vi "aproximateBall.vi"(6 "Radius":dbl, 8 "error in (no error)":errorcluster, 9 "Ball":refnum<class "Ball.lvclass">, 10 "Robot":refnum<class "Robot.lvclass">, 11 "KickToSkill in":refnum<class "KickToSkill.lvclass">) -> (0 "error out":errorcluster, 2 "Robot out":refnum<class "Robot.lvclass">, 3 "KickToSkill out":refnum<class "KickToSkill.lvclass">)   [LabVIEW 2023, in "KickToSkill.lvclass"]
uses:
  KickToSkill.lvclass
  Ball_class/Ball.lvclass
  C:/Users/lucio/Desktop/roboime/SSL_AI/Object_class/Object.lvclass
  Robot_class/Robot.lvclass
  Object_class/Object.lvclass/Object.ctl
  Robot_class/Robot.lvclass/Robot.ctl
  <vilib>/Analysis/baseanly.llb/Unit Vector (DBL).vi
  Object_class/Read position(x,y).vi
  Robot_class/Write dest_x.vi
  Robot_class/Write dest_y.vi
  Robot_class/Write dest_orientation.vi
  Utilities_class/Utilities.lvclass
  <vilib>/Analysis/NI_AALBase.lvlib
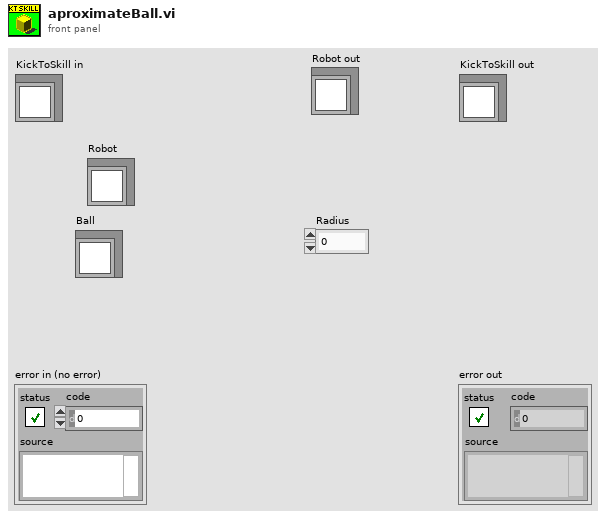
[diagram p1: front panel]
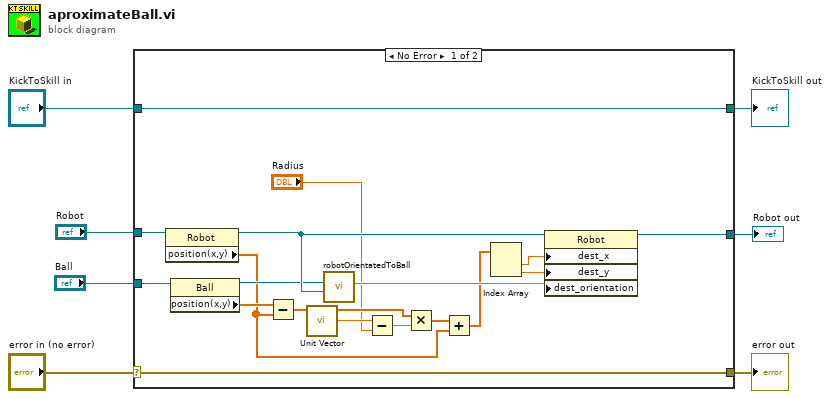
[diagram p0: block diagram]
diagram:
  n1 = case shown="No Error" "error in (no error)" {
    selector: "error in (no error)" -> [w25 w29]
    tunnel: [w25 w29] -> w6
    tunnel: [w26 w28] -> w4
    tunnel: "KickToSkill in" -> [w26 w28]
    tunnel: "Robot" -> [w23 w27]
    tunnel: "Ball" -> [w21 _]
    tunnel: [w9 w27] -> w1
    frame No Error {
      n2 = property class="Robot"(reference=w23) -> (reference out=w22:refnum<class "Robot.lvclass">, "position(x,y)"=w13:dbl[])  [unwired: 1 in, 1 out]
      n3 = property class="Ball"(reference=w21) -> (reference out=w20:refnum<class "Ball.lvclass">, "position(x,y)"=w19:dbl[])  [unwired: 1 in, 1 out]
      n4 = Subtract(x=w19, y=w13) -> (x-y=w18:dbl[])
      n5 = call-poly <vilib>:"Unit Vector.vi"("Input Vector"=w18) -> ("norm"=w17:dbl, "Unit Vector"=w15:dbl[])  [unwired: 8 in, 1 out]
      n6 = call "robotOrientatedToBall.vi"("Robot"=w22, "BallRef"=w20) -> ("Orientation"=w24:dbl)  [unwired: 7 in, 2 out]
      n7 = Subtract(x=w17, y="Radius") -> (x-y=w16:dbl)
      n8 = Multiply(x=w15, y=w16) -> (x*y=w14:dbl[])
      n9 = Add(x=w14, y=w13) -> (x+y=w12:dbl[])
      n10 = Index Array(array=w12) -> (element #1=w11:dbl, element #2=w10:dbl)  [unwired: 2 in]
      n11 = property class="Robot"(reference=w22, "dest_x"=w11, "dest_y"=w10, "dest_orientation"=w24) -> (reference out=w9:refnum<class "Robot.lvclass">)  [unwired: 1 in, 1 out]
    }
    frame Error {
    }
  }
  "error out" <- w6
  "KickToSkill out" <- w4
  "Robot out" <- w1
